vi "PH_HamamatsuCamera.constructor.vi"(0 "name":string, 2 "data in":string, 5 "error in(no error)":errorcluster) -> (14 "i ref out":refnum<vi>, 16 "data out":string, 19 "error out":errorcluster)   [LabVIEW 2014, in "PH_HamamatsuCamera.lvlib"]
doc: "This class controls a IEEE 1394 camera.\n\nThis class is part of the PHELIX user layer.\n\nauthor: Stefan Götte, GSI\n\nLicense Agreement for this software:\n\nCopyright (C)\nGesellschaft für Schwerionenforschung, GSI\nPlanckstr. 1\n64291 Darmstadt\nGermany\n\nContact: D.Beck@gsi.de \n\nThis program is free software; you can redistribute it and/or modify it under the terms of the \nGNU General Public License as published by the Free Software Foundation; either version 2 of \nthe license, or (at your option) any later version.\n\nThis program is distributed in the hope that it will be useful, but WITHOUT ANY WARRANTY; \nwithout even the implied warranty of MERCHANTABILITY or FITNESS FOR A PARTICULAR PURPOSE. See the GNU General License for more details (http://www.gnu.org).\n\nGesellschaft für Schwerionenforschung, GSI\nPlanckstr. 1, 64291 Darmstadt, Germany\nFor all questions and ideas contact: M.Richter@gsi.de, H.Brand@gsi.de or D.Beck@gsi.de.\nLast update: 16-JUN-2004"
uses:
  PH_HamamatsuCamera.lvlib
  PH_Basics/PH_Cam_BaseClass/PH_Cam_BaseClass.lvlib
  PH_Basics/PH_Class/PH_Class.lvlib
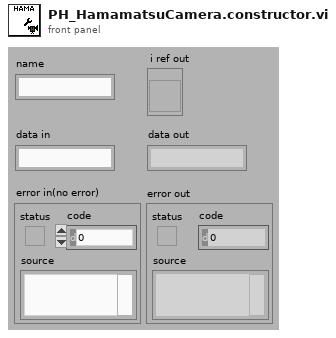
[diagram p1: front panel]
types:
  T1 = enum16{"SetAttribute", "GetAttribute", "CreateAttribute", "DestroyAttribute", "DestroyAllAtributes"}
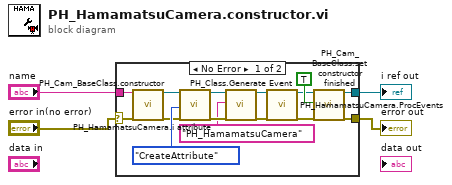
[diagram p0: block diagram]
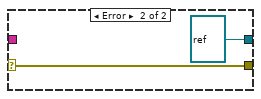
[diagram p2: hidden frame]
diagram:
  n1 = case shown="No Error" "error in(no error)" {
    selector: "error in(no error)" -> [w5 w21]
    tunnel: [w17 refnum<vi> refnum ("i ref out")] -> w4
    tunnel: [w18 w21] -> w3
    tunnel: "name" -> [w19 _]
    frame No Error {
      n2 = call "PH_Cam_BaseClass.constructor.vi"("name"=w19, "error in(no error)"=w5) -> ("i ref out"=w12:refnum<vi>, "error out"=w11:errorcluster)  [unwired: 15 in, 1 out]
      n3 = call "PH_HamamatsuCamera.i attribute.vi"("VI Refnum"=w12, "Action"=T1."CreateAttribute", "error in (no error)"=w11) -> ("VI Refnum out"=w10:refnum<vi>, "error out"=w9:errorcluster)  [unwired: 14 in, 1 out]
      n4 = call "PH_Class.Generate Event.vi"("i ref in"=w10, "Class"="PH_HamamatsuCamera", "error in (no error)"=w9) -> ("i ref out"=w8:refnum<vi>, "error out"=w7:errorcluster)  [unwired: 15 in]
      n5 = call "PH_HamamatsuCamera.ProcEvents.vi"("i ref in"=w8, "error in"=w7) -> ("i ref out"=w15:refnum<vi>, "error out"=w14:errorcluster)  [unwired: 16 in]
      n6 = call "PH_Cam_BaseClass.set constructor finished.vi"("i ref in"=w15, "Contructor finished"=TRUE, "error in (no error)"=w14) -> ("i ref out"=w17:refnum<vi>, "error out"=w18:errorcluster)  [unwired: 15 in]
    }
    frame Error {
    }
  }
  "i ref out" <- w4
  "error out" <- w3
